vi "load.vi"(5 "Python path":string="E:\\Python34\\python.exe", 7 "lvapi.py path":string="E:/Users/administrator/Documents/Python/dbm/LVAPI/lvapi.py", 8 "error in (no error)":errorcluster, 9 "ID":i32=1, 10 "Measurement":string="test_measurement", 11 "dbm in":refnum<class "dbm.lvclass">) -> (0 "error out":errorcluster, 3 "dbm out":refnum<class "dbm.lvclass">)   [LabVIEW 2013, in "dbm.lvclass"]
uses:
  dbm.lvclass
  dbm.lvclass/dbm.ctl
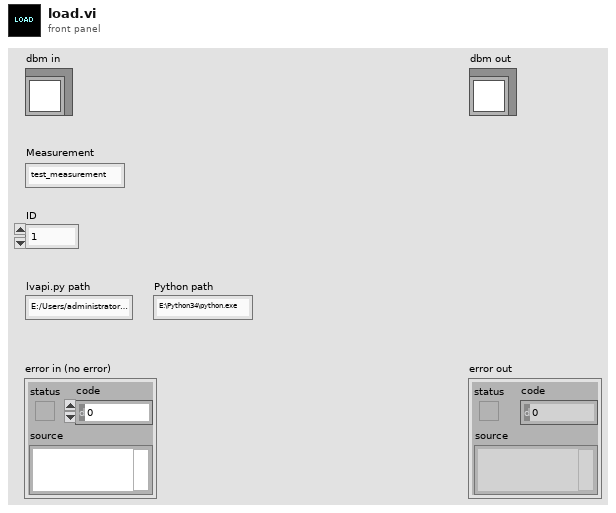
[diagram p1: front panel]
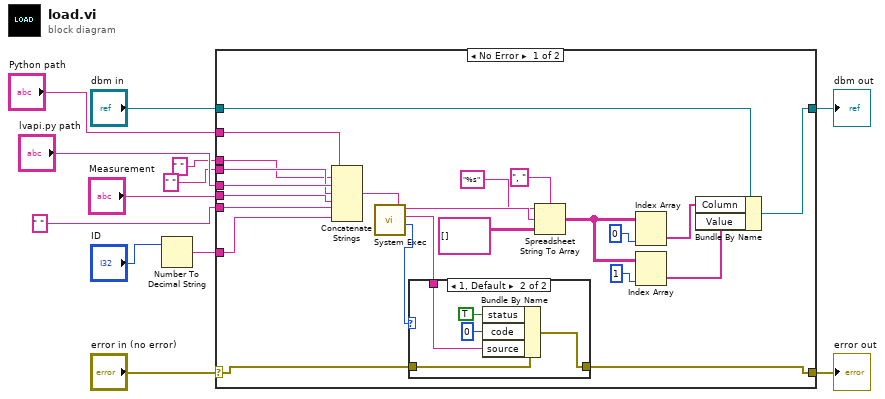
[diagram p0: block diagram]
diagram:
  n1 = Number To Decimal String(number="ID") -> (decimal integer string=w5:string)  [unwired: 1 in]
  n2 = case shown="No Error" "error in (no error)" {
    selector: "error in (no error)" -> [w22 w43]
    tunnel: [w21 w43] -> w11
    tunnel: [w27 w42] -> w9
    tunnel: "dbm in" -> [w28 w42]
    tunnel: "lvapi.py path" -> [w35 _]
    tunnel: "Measurement" -> [w16 _]
    tunnel: " " ("string") -> [w17 _]
    tunnel: w5 -> [w18 _]
    tunnel: " " ("string") -> [w15 _]
    tunnel: "Python path" -> [w14 _]
    tunnel: " " ("string") -> [w13 _]
    frame No Error {
      n3 = Concatenate Strings(w14, w13, w35, w15, w16, w17, w18) -> (w34:string)
      n4 = call <vilib>:"System Exec.vi"("command line"=w34) -> ("return code"=w19:i32, "standard error"=w20:string, "standard output"=w31:string)  [unwired: 7 in, 1 out]
      n5 = case shown="1, Default" w19 {
        tunnel: w22 -> [w36 w40]
        tunnel: [w36 w41] -> w21
        tunnel: w20 -> [_ w37]
        frame 0 {
        }
        frame 1, Default {
          n6 = Bundle By Name(cluster=w40, "status"=TRUE, "code"=0, "source"=w37) -> (w41:errorcluster)
        }
      }
      n7 = Spreadsheet String To Array(delimiter (Tab)=", ", format string="%s", spreadsheet string=w31, array type (2D Dbl)=string[][] []) -> (array=w29:string[][])
      n8 = Index Array(array=w29, index (col)=0 ("index (row)")) -> (element=w26:string[])  [unwired: 1 in]
      n9 = Index Array(array=w29, index (col)=1 ("index (row)")) -> (element=w25:string[])  [unwired: 1 in]
      n10 = Bundle By Name(cluster=w28, "Column"=w26, "Value"=w25) -> (w27:refnum<class "dbm.lvclass">)
    }
    frame Error {
    }
  }
  "error out" <- w11
  "dbm out" <- w9
